vi "Phase 3 Sequence Struct.vi"() -> ()   [LabVIEW 2017]
uses:
  Classes/Sequence/SequenceSubvis/TestStepTypes.ctl
  Classes/Sequence/SequenceSubvis/PolarizationSelect.ctl
  Classes/Sequence/SequenceSubvis/RF Direction.ctl
  Classes/Sequence/SequenceSubvis/TestStep-StepType.ctl
panel:
  out "test sequence in the new struct":T3(array[cluster])=[{"StepType"=enum."Patch", "RF In/Out"=enum."Tx - RF In", "Module/Raster"=0, "Polarization"=enum."Vertical", "PhaseShift deg"=[], "Attenuation dB"=[], "Position"={"X mm"=204.374756, "Y mm"=144.119598, "Z mm"=0.0, "T deg"=1.0}, "Patch RF In/Out"=TRUE}, {"StepType"=enum."SweepTest", "RF In/Out"=enum."Tx - RF In", "Module/Raster"=0, "Polarization"=enum."Vertical", "PhaseShift deg"=[0.0, 5.625, 11.25, 16.875, 22.5, 28.125, 33.75, 39.375, 45.0], "Attenuation dB"=[5.5], "Position"={"X mm"=204.374756, "Y mm"=144.119598, "Z mm"=0.0, "T deg"=1.0}, "Patch RF In/Out"=FALSE}, {"StepType"=enum."Patch", "RF In/Out"=enum."Tx - RF In", "Module/Raster"=0, "Polarization"=enum."Horizontal", "PhaseShift deg"=[], "Attenuation dB"=[], "Position"={"X mm"=204.374756, "Y mm"=144.119598, "Z mm"=0.0, "T deg"=1.0}, "Patch RF In/Out"=FALSE}, {"StepType"=enum."SweepTest", "RF In/Out"=enum."Tx - RF In", "Module/Raster"=0, "Polarization"=enum."Horizontal", "PhaseShift deg"=[0.0, 5.625, 11.25, 16.875, 22.5, 28.125, 33.75, 39.375, 45.0], "Attenuation dB"=[5.5], "Position"={"X mm"=204.374756, "Y mm"=144.119598, "Z mm"=0.0, "T deg"=1.0}, "Patch RF In/Out"=FALSE}, {"StepType"=enum."Patch", "RF In/Out"=enum."Tx - RF In", "Module/Raster"=1, "Polarization"=enum."Vertical", "PhaseShift deg"=[], "Attenuation dB"=[], "Position"={"X mm"=232.088571, "Y mm"=144.281169, "Z mm"=0.0, "T deg"=1.0}, "Patch RF In/Out"=FALSE}, {"StepType"=enum."SweepTest", "RF In/Out"=enum."Tx - RF In", "Module/Raster"=1, "Polarization"=enum."Vertical", "PhaseShift deg"=[90.0, 95.625, 101.25, 106.875, 112.5], "Attenuation dB"=[0.0, 0.5, 1.0, 1.5, 2.0, 2.5, 3.0, 3.5, 4.0, 4.5, 5.0, 5.5, 6.0, 6.5, 7.0, 7.5, 8.0, 8.5], "Position"={"X mm"=232.088571, "Y mm"=144.281169, "Z mm"=0.0, "T deg"=1.0}, "Patch RF In/Out"=FALSE}, {"StepType"=enum."Patch", "RF In/Out"=enum."Tx - RF In", "Module/Raster"=2, "Polarization"=enum."Vertical", "PhaseShift deg"=[], "Attenuation dB"=[], "Position"={"X mm"=259.802385, "Y mm"=144.442739, "Z mm"=0.0, "T deg"=1.0}, "Patch RF In/Out"=FALSE}, {"StepType"=enum."SweepTest", "RF In/Out"=enum."Tx - RF In", "Module/Raster"=2, "Polarization"=enum."Vertical", "PhaseShift deg"=[11.25, 16.875, 22.5, 28.125, 33.75, 39.375, 45.0, 50.625, 56.25, 61.875, 67.5, 73.125, 78.75, 84.375, 90.0, 95.625, 101.25, 106.875, 112.5], "Attenuation dB"=[0.0, 5.5, 7.0, 8.0, 9.0, 9.5], "Position"={"X mm"=259.802385, "Y mm"=144.442739, "Z mm"=0.0, "T deg"=1.0}, "Patch RF In/Out"=FALSE}, {"StepType"=enum."Patch", "RF In/Out"=enum."Tx - RF In", "Module/Raster"=15, "Polarization"=enum."Vertical", "PhaseShift deg"=[], "Attenuation dB"=[], "Position"={"X mm"=398.209889, "Y mm"=172.964406, "Z mm"=0.0, "T deg"=1.0}, "Patch RF In/Out"=FALSE}, {"StepType"=enum."SweepTest", "RF In/Out"=enum."Tx - RF In", "Module/Raster"=15, "Polarization"=enum."Vertical", "PhaseShift deg"=[0.0, 5.625, 11.25, 16.875, 22.5], "Attenuation dB"=[0.0, 0.5, 1.0, 1.5, 2.0], "Position"={"X mm"=398.209889, "Y mm"=172.964406, "Z mm"=0.0, "T deg"=1.0}, "Patch RF In/Out"=FALSE}, {"StepType"=enum."Patch", "RF In/Out"=enum."Tx - RF In", "Module/Raster"=17, "Polarization"=enum."Vertical", "PhaseShift deg"=[], "Attenuation dB"=[], "Position"={"X mm"=231.76543, "Y mm"=199.708798, "Z mm"=0.0, "T deg"=1.0}, "Patch RF In/Out"=FALSE}, {"StepType"=enum."SweepTest", "RF In/Out"=enum."Tx - RF In", "Module/Raster"=17, "Polarization"=enum."Vertical", "PhaseShift deg"=[0.0, 5.625], "Attenuation dB"=[0.0, 0.5], "Position"={"X mm"=231.76543, "Y mm"=199.708798, "Z mm"=0.0, "T deg"=1.0}, "Patch RF In/Out"=FALSE}, {"StepType"=enum."Patch", "RF In/Out"=enum."Tx - RF In", "Module/Raster"=21, "Polarization"=enum."Vertical", "PhaseShift deg"=[], "Attenuation dB"=[], "Position"={"X mm"=342.620689, "Y mm"=200.35508, "Z mm"=0.0, "T deg"=1.0}, "Patch RF In/Out"=FALSE}, {"StepType"=enum."SweepTest", "RF In/Out"=enum."Tx - RF In", "Module/Raster"=21, "Polarization"=enum."Vertical", "PhaseShift deg"=[0.0], "Attenuation dB"=[0.0], "Position"={"X mm"=342.620689, "Y mm"=200.35508, "Z mm"=0.0, "T deg"=1.0}, "Patch RF In/Out"=FALSE}, {"StepType"=enum."Patch", "RF In/Out"=enum."Tx - RF In", "Module/Raster"=23, "Polarization"=enum."Vertical", "PhaseShift deg"=[], "Attenuation dB"=[], "Position"={"X mm"=398.048318, "Y mm"=200.678221, "Z mm"=0.0, "T deg"=1.0}, "Patch RF In/Out"=FALSE}, {"StepType"=enum."SweepTest", "RF In/Out"=enum."Tx - RF In", "Module/Raster"=23, "Polarization"=enum."Vertical", "PhaseShift deg"=[0.0], "Attenuation dB"=[0.0], "Position"={"X mm"=398.048318, "Y mm"=200.678221, "Z mm"=0.0, "T deg"=1.0}, "Patch RF In/Out"=FALSE}, {"StepType"=enum."Patch", "RF In/Out"=enum."Tx - RF In", "Module/Raster"=24, "Polarization"=enum."Vertical", "PhaseShift deg"=[], "Attenuation dB"=[], "Position"={"X mm"=203.890045, "Y mm"=227.261043, "Z mm"=0.0, "T deg"=1.0}, "Patch RF In/Out"=FALSE}, {"StepType"=enum."SweepTest", "RF In/Out"=enum."Tx - RF In", "Module/Raster"=24, "Polarization"=enum."Vertical", "PhaseShift deg"=[0.0, 5.625, 11.25], "Attenuation dB"=[0.0], "Position"={"X mm"=203.890045, "Y mm"=227.261043, "Z mm"=0.0, "T deg"=1.0}, "Patch RF In/Out"=FALSE}, {"StepType"=enum."Patch", "RF In/Out"=enum."Tx - RF In", "Module/Raster"=25, "Polarization"=enum."Vertical", "PhaseShift deg"=[], "Attenuation dB"=[], "Position"={"X mm"=231.603859, "Y mm"=227.422613, "Z mm"=0.0, "T deg"=1.0}, "Patch RF In/Out"=FALSE}, {"StepType"=enum."SweepTest", "RF In/Out"=enum."Tx - RF In", "Module/Raster"=25, "Polarization"=enum."Vertical", "PhaseShift deg"=[0.0], "Attenuation dB"=[0.0], "Position"={"X mm"=231.603859, "Y mm"=227.422613, "Z mm"=0.0, "T deg"=1.0}, "Patch RF In/Out"=FALSE}, {"StepType"=enum."Patch", "RF In/Out"=enum."Tx - RF In", "Module/Raster"=31, "Polarization"=enum."Vertical", "PhaseShift deg"=[], "Attenuation dB"=[], "Position"={"X mm"=397.886748, "Y mm"=228.392036, "Z mm"=0.0, "T deg"=1.0}, "Patch RF In/Out"=FALSE}, {"StepType"=enum."SweepTest", "RF In/Out"=enum."Tx - RF In", "Module/Raster"=31, "Polarization"=enum."Vertical", "PhaseShift deg"=[0.0, 5.625], "Attenuation dB"=[0.0], "Position"={"X mm"=397.886748, "Y mm"=228.392036, "Z mm"=0.0, "T deg"=1.0}, "Patch RF In/Out"=FALSE}, {"StepType"=enum."Patch", "RF In/Out"=enum."Tx - RF In", "Module/Raster"=31, "Polarization"=enum."Horizontal", "PhaseShift deg"=[], "Attenuation dB"=[], "Position"={"X mm"=397.886748, "Y mm"=228.392036, "Z mm"=0.0, "T deg"=1.0}, "Patch RF In/Out"=FALSE}, {"StepType"=enum."SweepTest", "RF In/Out"=enum."Tx - RF In", "Module/Raster"=31, "Polarization"=enum."Horizontal", "PhaseShift deg"=[0.0, 5.625], "Attenuation dB"=[0.0], "Position"={"X mm"=397.886748, "Y mm"=228.392036, "Z mm"=0.0, "T deg"=1.0}, "Patch RF In/Out"=FALSE}, {"StepType"=enum."Patch", "RF In/Out"=enum."Tx - RF In", "Module/Raster"=39, "Polarization"=enum."Vertical", "PhaseShift deg"=[], "Attenuation dB"=[], "Position"={"X mm"=397.725177, "Y mm"=256.10585, "Z mm"=0.0, "T deg"=1.0}, "Patch RF In/Out"=FALSE}, {"StepType"=enum."SweepTest", "RF In/Out"=enum."Tx - RF In", "Module/Raster"=39, "Polarization"=enum."Vertical", "PhaseShift deg"=[0.0], "Attenuation dB"=[0.0], "Position"={"X mm"=397.725177, "Y mm"=256.10585, "Z mm"=0.0, "T deg"=1.0}, "Patch RF In/Out"=FALSE}, {"StepType"=enum."Patch", "RF In/Out"=enum."Tx - RF In", "Module/Raster"=44, "Polarization"=enum."Vertical", "PhaseShift deg"=[], "Attenuation dB"=[], "Position"={"X mm"=314.422163, "Y mm"=283.334954, "Z mm"=0.0, "T deg"=1.0}, "Patch RF In/Out"=FALSE}, {"StepType"=enum."SweepTest", "RF In/Out"=enum."Tx - RF In", "Module/Raster"=44, "Polarization"=enum."Vertical", "PhaseShift deg"=[0.0, 5.625], "Attenuation dB"=[0.0, 0.5], "Position"={"X mm"=314.422163, "Y mm"=283.334954, "Z mm"=0.0, "T deg"=1.0}, "Patch RF In/Out"=FALSE}, {"StepType"=enum."Patch", "RF In/Out"=enum."Tx - RF In", "Module/Raster"=45, "Polarization"=enum."Vertical", "PhaseShift deg"=[], "Attenuation dB"=[], "Position"={"X mm"=342.135977, "Y mm"=283.496524, "Z mm"=0.0, "T deg"=1.0}, "Patch RF In/Out"=FALSE}, {"StepType"=enum."SweepTest", "RF In/Out"=enum."Tx - RF In", "Module/Raster"=45, "Polarization"=enum."Vertical", "PhaseShift deg"=[0.0], "Attenuation dB"=[0.0], "Position"={"X mm"=342.135977, "Y mm"=283.496524, "Z mm"=0.0, "T deg"=1.0}, "Patch RF In/Out"=FALSE}, {"StepType"=enum."Patch", "RF In/Out"=enum."Tx - RF In", "Module/Raster"=46, "Polarization"=enum."Vertical", "PhaseShift deg"=[], "Attenuation dB"=[], "Position"={"X mm"=369.849792, "Y mm"=283.658095, "Z mm"=0.0, "T deg"=1.0}, "Patch RF In/Out"=FALSE}, {"StepType"=enum."SweepTest", "RF In/Out"=enum."Tx - RF In", "Module/Raster"=46, "Polarization"=enum."Vertical", "PhaseShift deg"=[0.0, 5.625], "Attenuation dB"=[0.0, 0.5], "Position"={"X mm"=369.849792, "Y mm"=283.658095, "Z mm"=0.0, "T deg"=1.0}, "Patch RF In/Out"=FALSE}, {"StepType"=enum."Patch", "RF In/Out"=enum."Tx - RF In", "Module/Raster"=47, "Polarization"=enum."Vertical", "PhaseShift deg"=[], "Attenuation dB"=[], "Position"={"X mm"=397.563607, "Y mm"=283.819665, "Z mm"=0.0, "T deg"=1.0}, "Patch RF In/Out"=FALSE}, {"StepType"=enum."SweepTest", "RF In/Out"=enum."Tx - RF In", "Module/Raster"=47, "Polarization"=enum."Vertical", "PhaseShift deg"=[0.0], "Attenuation dB"=[0.0], "Position"={"X mm"=397.563607, "Y mm"=283.819665, "Z mm"=0.0, "T deg"=1.0}, "Patch RF In/Out"=FALSE}, {"StepType"=enum."Patch", "RF In/Out"=enum."Tx - RF In", "Module/Raster"=48, "Polarization"=enum."Vertical", "PhaseShift deg"=[], "Attenuation dB"=[], "Position"={"X mm"=203.405333, "Y mm"=310.402487, "Z mm"=0.0, "T deg"=1.0}, "Patch RF In/Out"=FALSE}, {"StepType"=enum."SweepTest", "RF In/Out"=enum."Tx - RF In", "Module/Raster"=48, "Polarization"=enum."Vertical", "PhaseShift deg"=[28.125], "Attenuation dB"=[2.5], "Position"={"X mm"=203.405333, "Y mm"=310.402487, "Z mm"=0.0, "T deg"=1.0}, "Patch RF In/Out"=FALSE}, {"StepType"=enum."Patch", "RF In/Out"=enum."Tx - RF In", "Module/Raster"=48, "Polarization"=enum."Horizontal", "PhaseShift deg"=[], "Attenuation dB"=[], "Position"={"X mm"=203.405333, "Y mm"=310.402487, "Z mm"=0.0, "T deg"=1.0}, "Patch RF In/Out"=FALSE}, {"StepType"=enum."SweepTest", "RF In/Out"=enum."Tx - RF In", "Module/Raster"=48, "Polarization"=enum."Horizontal", "PhaseShift deg"=[28.125], "Attenuation dB"=[2.5], "Position"={"X mm"=203.405333, "Y mm"=310.402487, "Z mm"=0.0, "T deg"=1.0}, "Patch RF In/Out"=FALSE}, {"StepType"=enum."Patch", "RF In/Out"=enum."Tx - RF In", "Module/Raster"=55, "Polarization"=enum."Vertical", "PhaseShift deg"=[], "Attenuation dB"=[], "Position"={"X mm"=397.402037, "Y mm"=311.53348, "Z mm"=0.0, "T deg"=1.0}, "Patch RF In/Out"=FALSE}, {"StepType"=enum."SweepTest", "RF In/Out"=enum."Tx - RF In", "Module/Raster"=55, "Polarization"=enum."Vertical", "PhaseShift deg"=[0.0, 5.625, 11.25, 16.875, 22.5], "Attenuation dB"=[0.0, 0.5, 1.0], "Position"={"X mm"=397.402037, "Y mm"=311.53348, "Z mm"=0.0, "T deg"=1.0}, "Patch RF In/Out"=FALSE}, {"StepType"=enum."Patch", "RF In/Out"=enum."Tx - RF In", "Module/Raster"=59, "Polarization"=enum."Vertical", "PhaseShift deg"=[], "Attenuation dB"=[], "Position"={"X mm"=286.385207, "Y mm"=338.601013, "Z mm"=0.0, "T deg"=1.0}, "Patch RF In/Out"=FALSE}, {"StepType"=enum."SweepTest", "RF In/Out"=enum."Tx - RF In", "Module/Raster"=59, "Polarization"=enum."Vertical", "PhaseShift deg"=[0.0], "Attenuation dB"=[0.0], "Position"={"X mm"=286.385207, "Y mm"=338.601013, "Z mm"=0.0, "T deg"=1.0}, "Patch RF In/Out"=FALSE}, {"StepType"=enum."Patch", "RF In/Out"=enum."Tx - RF In", "Module/Raster"=59, "Polarization"=enum."Horizontal", "PhaseShift deg"=[], "Attenuation dB"=[], "Position"={"X mm"=286.385207, "Y mm"=338.601013, "Z mm"=0.0, "T deg"=1.0}, "Patch RF In/Out"=FALSE}, {"StepType"=enum."SweepTest", "RF In/Out"=enum."Tx - RF In", "Module/Raster"=59, "Polarization"=enum."Horizontal", "PhaseShift deg"=[0.0], "Attenuation dB"=[0.0], "Position"={"X mm"=286.385207, "Y mm"=338.601013, "Z mm"=0.0, "T deg"=1.0}, "Patch RF In/Out"=FALSE}, {"StepType"=enum."Patch", "RF In/Out"=enum."Tx - RF In", "Module/Raster"=62, "Polarization"=enum."Vertical", "PhaseShift deg"=[], "Attenuation dB"=[], "Position"={"X mm"=369.526651, "Y mm"=339.085724, "Z mm"=0.0, "T deg"=1.0}, "Patch RF In/Out"=FALSE}, {"StepType"=enum."SweepTest", "RF In/Out"=enum."Tx - RF In", "Module/Raster"=62, "Polarization"=enum."Vertical", "PhaseShift deg"=[0.0, 5.625, 11.25, 16.875, 22.5, 28.125], "Attenuation dB"=[0.0, 0.5, 1.0, 1.5, 2.0, 2.5], "Position"={"X mm"=369.526651, "Y mm"=339.085724, "Z mm"=0.0, "T deg"=1.0}, "Patch RF In/Out"=FALSE}, {"StepType"=enum."Patch", "RF In/Out"=enum."Tx - RF In", "Module/Raster"=63, "Polarization"=enum."Vertical", "PhaseShift deg"=[], "Attenuation dB"=[], "Position"={"X mm"=397.240466, "Y mm"=339.247295, "Z mm"=0.0, "T deg"=1.0}, "Patch RF In/Out"=FALSE}, {"StepType"=enum."SweepTest", "RF In/Out"=enum."Tx - RF In", "Module/Raster"=63, "Polarization"=enum."Vertical", "PhaseShift deg"=[0.0, 5.625, 11.25, 16.875, 22.5, 28.125], "Attenuation dB"=[0.0, 0.5, 1.0, 1.5, 2.0, 2.5], "Position"={"X mm"=397.240466, "Y mm"=339.247295, "Z mm"=0.0, "T deg"=1.0}, "Patch RF In/Out"=FALSE}, {"StepType"=enum."Patch", "RF In/Out"=enum."Rx - RF Out", "Module/Raster"=0, "Polarization"=enum."Vertical", "PhaseShift deg"=[], "Attenuation dB"=[], "Position"={"X mm"=204.374756, "Y mm"=144.119598, "Z mm"=0.0, "T deg"=1.0}, "Patch RF In/Out"=TRUE}, {"StepType"=enum."SweepTest", "RF In/Out"=enum."Rx - RF Out", "Module/Raster"=0, "Polarization"=enum."Vertical", "PhaseShift deg"=[0.0, 5.625, 11.25, 16.875, 22.5, 28.125, 33.75, 39.375, 45.0], "Attenuation dB"=[5.5], "Position"={"X mm"=204.374756, "Y mm"=144.119598, "Z mm"=0.0, "T deg"=1.0}, "Patch RF In/Out"=FALSE}, {"StepType"=enum."Patch", "RF In/Out"=enum."Rx - RF Out", "Module/Raster"=0, "Polarization"=enum."Horizontal", "PhaseShift deg"=[], "Attenuation dB"=[], "Position"={"X mm"=204.374756, "Y mm"=144.119598, "Z mm"=0.0, "T deg"=1.0}, "Patch RF In/Out"=FALSE}, {"StepType"=enum."SweepTest", "RF In/Out"=enum."Rx - RF Out", "Module/Raster"=0, "Polarization"=enum."Horizontal", "PhaseShift deg"=[0.0, 5.625, 11.25, 16.875, 22.5, 28.125, 33.75, 39.375, 45.0], "Attenuation dB"=[5.5], "Position"={"X mm"=204.374756, "Y mm"=144.119598, "Z mm"=0.0, "T deg"=1.0}, "Patch RF In/Out"=FALSE}, {"StepType"=enum."Patch", "RF In/Out"=enum."Rx - RF Out", "Module/Raster"=17, "Polarization"=enum."Horizontal", "PhaseShift deg"=[], "Attenuation dB"=[], "Position"={"X mm"=231.76543, "Y mm"=199.708798, "Z mm"=0.0, "T deg"=1.0}, "Patch RF In/Out"=FALSE}, {"StepType"=enum."SweepTest", "RF In/Out"=enum."Rx - RF Out", "Module/Raster"=17, "Polarization"=enum."Horizontal", "PhaseShift deg"=[0.0, 5.625], "Attenuation dB"=[0.0, 0.5], "Position"={"X mm"=231.76543, "Y mm"=199.708798, "Z mm"=0.0, "T deg"=1.0}, "Patch RF In/Out"=FALSE}, {"StepType"=enum."Patch", "RF In/Out"=enum."Rx - RF Out", "Module/Raster"=28, "Polarization"=enum."Vertical", "PhaseShift deg"=[], "Attenuation dB"=[], "Position"={"X mm"=314.745304, "Y mm"=227.907324, "Z mm"=0.0, "T deg"=1.0}, "Patch RF In/Out"=FALSE}, {"StepType"=enum."SweepTest", "RF In/Out"=enum."Rx - RF Out", "Module/Raster"=28, "Polarization"=enum."Vertical", "PhaseShift deg"=[0.0], "Attenuation dB"=[0.0], "Position"={"X mm"=314.745304, "Y mm"=227.907324, "Z mm"=0.0, "T deg"=1.0}, "Patch RF In/Out"=FALSE}, {"StepType"=enum."Patch", "RF In/Out"=enum."Rx - RF Out", "Module/Raster"=28, "Polarization"=enum."Horizontal", "PhaseShift deg"=[], "Attenuation dB"=[], "Position"={"X mm"=314.745304, "Y mm"=227.907324, "Z mm"=0.0, "T deg"=1.0}, "Patch RF In/Out"=FALSE}, {"StepType"=enum."SweepTest", "RF In/Out"=enum."Rx - RF Out", "Module/Raster"=28, "Polarization"=enum."Horizontal", "PhaseShift deg"=[0.0], "Attenuation dB"=[0.0], "Position"={"X mm"=314.745304, "Y mm"=227.907324, "Z mm"=0.0, "T deg"=1.0}, "Patch RF In/Out"=FALSE}, {"StepType"=enum."Patch", "RF In/Out"=enum."Rx - RF Out", "Module/Raster"=31, "Polarization"=enum."Vertical", "PhaseShift deg"=[], "Attenuation dB"=[], "Position"={"X mm"=397.886748, "Y mm"=228.392036, "Z mm"=0.0, "T deg"=1.0}, "Patch RF In/Out"=FALSE}, {"StepType"=enum."SweepTest", "RF In/Out"=enum."Rx - RF Out", "Module/Raster"=31, "Polarization"=enum."Vertical", "PhaseShift deg"=[0.0, 5.625], "Attenuation dB"=[0.0], "Position"={"X mm"=397.886748, "Y mm"=228.392036, "Z mm"=0.0, "T deg"=1.0}, "Patch RF In/Out"=FALSE}, {"StepType"=enum."Patch", "RF In/Out"=enum."Rx - RF Out", "Module/Raster"=31, "Polarization"=enum."Horizontal", "PhaseShift deg"=[], "Attenuation dB"=[], "Position"={"X mm"=397.886748, "Y mm"=228.392036, "Z mm"=0.0, "T deg"=1.0}, "Patch RF In/Out"=FALSE}, {"StepType"=enum."SweepTest", "RF In/Out"=enum."Rx - RF Out", "Module/Raster"=31, "Polarization"=enum."Horizontal", "PhaseShift deg"=[0.0, 5.625], "Attenuation dB"=[0.0], "Position"={"X mm"=397.886748, "Y mm"=228.392036, "Z mm"=0.0, "T deg"=1.0}, "Patch RF In/Out"=FALSE}, {"StepType"=enum."Patch", "RF In/Out"=enum."Rx - RF Out", "Module/Raster"=36, "Polarization"=enum."Vertical", "PhaseShift deg"=[], "Attenuation dB"=[], "Position"={"X mm"=314.583733, "Y mm"=255.621139, "Z mm"=0.0, "T deg"=1.0}, "Patch RF In/Out"=FALSE}, {"StepType"=enum."SweepTest", "RF In/Out"=enum."Rx - RF Out", "Module/Raster"=36, "Polarization"=enum."Vertical", "PhaseShift deg"=[28.125, 33.75, 39.375, 45.0, 50.625], "Attenuation dB"=[5.0, 5.5, 6.0, 6.5, 7.0], "Position"={"X mm"=314.583733, "Y mm"=255.621139, "Z mm"=0.0, "T deg"=1.0}, "Patch RF In/Out"=FALSE}, {"StepType"=enum."Patch", "RF In/Out"=enum."Rx - RF Out", "Module/Raster"=36, "Polarization"=enum."Horizontal", "PhaseShift deg"=[], "Attenuation dB"=[], "Position"={"X mm"=314.583733, "Y mm"=255.621139, "Z mm"=0.0, "T deg"=1.0}, "Patch RF In/Out"=FALSE}, {"StepType"=enum."SweepTest", "RF In/Out"=enum."Rx - RF Out", "Module/Raster"=36, "Polarization"=enum."Horizontal", "PhaseShift deg"=[28.125, 33.75, 39.375, 45.0, 50.625], "Attenuation dB"=[5.0, 5.5, 6.0, 6.5, 7.0], "Position"={"X mm"=314.583733, "Y mm"=255.621139, "Z mm"=0.0, "T deg"=1.0}, "Patch RF In/Out"=FALSE}, {"StepType"=enum."Patch", "RF In/Out"=enum."Rx - RF Out", "Module/Raster"=48, "Polarization"=enum."Vertical", "PhaseShift deg"=[], "Attenuation dB"=[], "Position"={"X mm"=203.405333, "Y mm"=310.402487, "Z mm"=0.0, "T deg"=1.0}, "Patch RF In/Out"=FALSE}, {"StepType"=enum."SweepTest", "RF In/Out"=enum."Rx - RF Out", "Module/Raster"=48, "Polarization"=enum."Vertical", "PhaseShift deg"=[28.125], "Attenuation dB"=[2.5], "Position"={"X mm"=203.405333, "Y mm"=310.402487, "Z mm"=0.0, "T deg"=1.0}, "Patch RF In/Out"=FALSE}, {"StepType"=enum."Patch", "RF In/Out"=enum."Rx - RF Out", "Module/Raster"=48, "Polarization"=enum."Horizontal", "PhaseShift deg"=[], "Attenuation dB"=[], "Position"={"X mm"=203.405333, "Y mm"=310.402487, "Z mm"=0.0, "T deg"=1.0}, "Patch RF In/Out"=FALSE}, {"StepType"=enum."SweepTest", "RF In/Out"=enum."Rx - RF Out", "Module/Raster"=48, "Polarization"=enum."Horizontal", "PhaseShift deg"=[28.125], "Attenuation dB"=[2.5], "Position"={"X mm"=203.405333, "Y mm"=310.402487, "Z mm"=0.0, "T deg"=1.0}, "Patch RF In/Out"=FALSE}, {"StepType"=enum."Patch", "RF In/Out"=enum."Rx - RF Out", "Module/Raster"=59, "Polarization"=enum."Vertical", "PhaseShift deg"=[], "Attenuation dB"=[], "Position"={"X mm"=286.385207, "Y mm"=338.601013, "Z mm"=0.0, "T deg"=1.0}, "Patch RF In/Out"=FALSE}, {"StepType"=enum."SweepTest", "RF In/Out"=enum."Rx - RF Out", "Module/Raster"=59, "Polarization"=enum."Vertical", "PhaseShift deg"=[0.0], "Attenuation dB"=[0.0], "Position"={"X mm"=286.385207, "Y mm"=338.601013, "Z mm"=0.0, "T deg"=1.0}, "Patch RF In/Out"=FALSE}, {"StepType"=enum."Patch", "RF In/Out"=enum."Rx - RF Out", "Module/Raster"=59, "Polarization"=enum."Horizontal", "PhaseShift deg"=[], "Attenuation dB"=[], "Position"={"X mm"=286.385207, "Y mm"=338.601013, "Z mm"=0.0, "T deg"=1.0}, "Patch RF In/Out"=FALSE}, {"StepType"=enum."SweepTest", "RF In/Out"=enum."Rx - RF Out", "Module/Raster"=59, "Polarization"=enum."Horizontal", "PhaseShift deg"=[0.0], "Attenuation dB"=[0.0], "Position"={"X mm"=286.385207, "Y mm"=338.601013, "Z mm"=0.0, "T deg"=1.0}, "Patch RF In/Out"=FALSE}, {"StepType"=enum."Patch", "RF In/Out"=enum."Rx - RF Out", "Module/Raster"=62, "Polarization"=enum."Vertical", "PhaseShift deg"=[], "Attenuation dB"=[], "Position"={"X mm"=369.526651, "Y mm"=339.085724, "Z mm"=0.0, "T deg"=1.0}, "Patch RF In/Out"=FALSE}, {"StepType"=enum."SweepTest", "RF In/Out"=enum."Rx - RF Out", "Module/Raster"=62, "Polarization"=enum."Vertical", "PhaseShift deg"=[0.0, 5.625, 11.25, 16.875, 22.5, 28.125], "Attenuation dB"=[0.0, 0.5, 1.0, 1.5, 2.0, 2.5], "Position"={"X mm"=369.526651, "Y mm"=339.085724, "Z mm"=0.0, "T deg"=1.0}, "Patch RF In/Out"=FALSE}, {"StepType"=enum."Patch", "RF In/Out"=enum."Rx - RF Out", "Module/Raster"=63, "Polarization"=enum."Vertical", "PhaseShift deg"=[], "Attenuation dB"=[], "Position"={"X mm"=397.240466, "Y mm"=339.247295, "Z mm"=0.0, "T deg"=1.0}, "Patch RF In/Out"=FALSE}, {"StepType"=enum."SweepTest", "RF In/Out"=enum."Rx - RF Out", "Module/Raster"=63, "Polarization"=enum."Vertical", "PhaseShift deg"=[0.0, 5.625, 11.25, 16.875, 22.5, 28.125], "Attenuation dB"=[0.0, 0.5, 1.0, 1.5, 2.0, 2.5], "Position"={"X mm"=397.240466, "Y mm"=339.247295, "Z mm"=0.0, "T deg"=1.0}, "Patch RF In/Out"=FALSE}, {"StepType"=enum."Finish", "RF In/Out"=enum."Tx - RF In", "Module/Raster"=0, "Polarization"=enum."Vertical", "PhaseShift deg"=[], "Attenuation dB"=[], "Position"={"X mm"=204.374756, "Y mm"=144.119598, "Z mm"=0.0, "T deg"=1.0}, "Patch RF In/Out"=FALSE}]
  out "TestSequence New":T3(array[cluster])
  in  "Motion":bool
  in  "from Raster Test File":T4
  in  "Raster":bool
  in  "TestSequence":T5[](array[typedef])=[{"RF In/Out"=enum."Tx - RF In", "TR Module 0-7"=0, "Polarization"=enum."Vertical", "PhaseShift deg"=[], "Attenuation dB"=[], "StepType"=enum."NewConnection"}, {"RF In/Out"=enum."Tx - RF In", "TR Module 0-7"=0, "Polarization"=enum."Vertical", "PhaseShift deg"=[0.0, 5.625, 11.25, 16.875, 22.5, 28.125, 33.75, 39.375, 45.0], "Attenuation dB"=[5.5], "StepType"=enum."SweepTest"}, {"RF In/Out"=enum."Tx - RF In", "TR Module 0-7"=0, "Polarization"=enum."Horizontal", "PhaseShift deg"=[], "Attenuation dB"=[], "StepType"=enum."NewConnection"}, {"RF In/Out"=enum."Tx - RF In", "TR Module 0-7"=0, "Polarization"=enum."Horizontal", "PhaseShift deg"=[0.0, 5.625, 11.25, 16.875, 22.5, 28.125, 33.75, 39.375, 45.0], "Attenuation dB"=[5.5], "StepType"=enum."SweepTest"}, {"RF In/Out"=enum."Tx - RF In", "TR Module 0-7"=1, "Polarization"=enum."Vertical", "PhaseShift deg"=[], "Attenuation dB"=[], "StepType"=enum."NewConnection"}, {"RF In/Out"=enum."Tx - RF In", "TR Module 0-7"=1, "Polarization"=enum."Vertical", "PhaseShift deg"=[90.0, 95.625, 101.25, 106.875, 112.5], "Attenuation dB"=[0.0, 0.5, 1.0, 1.5, 2.0, 2.5, 3.0, 3.5, 4.0, 4.5, 5.0, 5.5, 6.0, 6.5, 7.0, 7.5, 8.0, 8.5], "StepType"=enum."SweepTest"}, {"RF In/Out"=enum."Tx - RF In", "TR Module 0-7"=2, "Polarization"=enum."Vertical", "PhaseShift deg"=[], "Attenuation dB"=[], "StepType"=enum."NewConnection"}, {"RF In/Out"=enum."Tx - RF In", "TR Module 0-7"=2, "Polarization"=enum."Vertical", "PhaseShift deg"=[11.25, 16.875, 22.5, 28.125, 33.75, 39.375, 45.0, 50.625, 56.25, 61.875, 67.5, 73.125, 78.75, 84.375, 90.0, 95.625, 101.25, 106.875, 112.5], "Attenuation dB"=[0.0, 5.5, 7.0, 8.0, 9.0, 9.5], "StepType"=enum."SweepTest"}, {"RF In/Out"=enum."Tx - RF In", "TR Module 0-7"=15, "Polarization"=enum."Vertical", "PhaseShift deg"=[], "Attenuation dB"=[], "StepType"=enum."NewConnection"}, {"RF In/Out"=enum."Tx - RF In", "TR Module 0-7"=15, "Polarization"=enum."Vertical", "PhaseShift deg"=[0.0, 5.625, 11.25, 16.875, 22.5], "Attenuation dB"=[0.0, 0.5, 1.0, 1.5, 2.0], "StepType"=enum."SweepTest"}, {"RF In/Out"=enum."Tx - RF In", "TR Module 0-7"=17, "Polarization"=enum."Vertical", "PhaseShift deg"=[], "Attenuation dB"=[], "StepType"=enum."NewConnection"}, {"RF In/Out"=enum."Tx - RF In", "TR Module 0-7"=17, "Polarization"=enum."Vertical", "PhaseShift deg"=[0.0, 5.625], "Attenuation dB"=[0.0, 0.5], "StepType"=enum."SweepTest"}, {"RF In/Out"=enum."Tx - RF In", "TR Module 0-7"=21, "Polarization"=enum."Vertical", "PhaseShift deg"=[], "Attenuation dB"=[], "StepType"=enum."NewConnection"}, {"RF In/Out"=enum."Tx - RF In", "TR Module 0-7"=21, "Polarization"=enum."Vertical", "PhaseShift deg"=[0.0], "Attenuation dB"=[0.0], "StepType"=enum."SweepTest"}, {"RF In/Out"=enum."Tx - RF In", "TR Module 0-7"=23, "Polarization"=enum."Vertical", "PhaseShift deg"=[], "Attenuation dB"=[], "StepType"=enum."NewConnection"}, {"RF In/Out"=enum."Tx - RF In", "TR Module 0-7"=23, "Polarization"=enum."Vertical", "PhaseShift deg"=[0.0], "Attenuation dB"=[0.0], "StepType"=enum."SweepTest"}, {"RF In/Out"=enum."Tx - RF In", "TR Module 0-7"=24, "Polarization"=enum."Vertical", "PhaseShift deg"=[], "Attenuation dB"=[], "StepType"=enum."NewConnection"}, {"RF In/Out"=enum."Tx - RF In", "TR Module 0-7"=24, "Polarization"=enum."Vertical", "PhaseShift deg"=[0.0, 5.625, 11.25], "Attenuation dB"=[0.0], "StepType"=enum."SweepTest"}, {"RF In/Out"=enum."Tx - RF In", "TR Module 0-7"=25, "Polarization"=enum."Vertical", "PhaseShift deg"=[], "Attenuation dB"=[], "StepType"=enum."NewConnection"}, {"RF In/Out"=enum."Tx - RF In", "TR Module 0-7"=25, "Polarization"=enum."Vertical", "PhaseShift deg"=[0.0], "Attenuation dB"=[0.0], "StepType"=enum."SweepTest"}, {"RF In/Out"=enum."Tx - RF In", "TR Module 0-7"=31, "Polarization"=enum."Vertical", "PhaseShift deg"=[], "Attenuation dB"=[], "StepType"=enum."NewConnection"}, {"RF In/Out"=enum."Tx - RF In", "TR Module 0-7"=31, "Polarization"=enum."Vertical", "PhaseShift deg"=[0.0, 5.625], "Attenuation dB"=[0.0], "StepType"=enum."SweepTest"}, {"RF In/Out"=enum."Tx - RF In", "TR Module 0-7"=31, "Polarization"=enum."Horizontal", "PhaseShift deg"=[], "Attenuation dB"=[], "StepType"=enum."NewConnection"}, {"RF In/Out"=enum."Tx - RF In", "TR Module 0-7"=31, "Polarization"=enum."Horizontal", "PhaseShift deg"=[0.0, 5.625], "Attenuation dB"=[0.0], "StepType"=enum."SweepTest"}, {"RF In/Out"=enum."Tx - RF In", "TR Module 0-7"=39, "Polarization"=enum."Vertical", "PhaseShift deg"=[], "Attenuation dB"=[], "StepType"=enum."NewConnection"}, {"RF In/Out"=enum."Tx - RF In", "TR Module 0-7"=39, "Polarization"=enum."Vertical", "PhaseShift deg"=[0.0], "Attenuation dB"=[0.0], "StepType"=enum."SweepTest"}, {"RF In/Out"=enum."Tx - RF In", "TR Module 0-7"=44, "Polarization"=enum."Vertical", "PhaseShift deg"=[], "Attenuation dB"=[], "StepType"=enum."NewConnection"}, {"RF In/Out"=enum."Tx - RF In", "TR Module 0-7"=44, "Polarization"=enum."Vertical", "PhaseShift deg"=[0.0, 5.625], "Attenuation dB"=[0.0, 0.5], "StepType"=enum."SweepTest"}, {"RF In/Out"=enum."Tx - RF In", "TR Module 0-7"=45, "Polarization"=enum."Vertical", "PhaseShift deg"=[], "Attenuation dB"=[], "StepType"=enum."NewConnection"}, {"RF In/Out"=enum."Tx - RF In", "TR Module 0-7"=45, "Polarization"=enum."Vertical", "PhaseShift deg"=[0.0], "Attenuation dB"=[0.0], "StepType"=enum."SweepTest"}, {"RF In/Out"=enum."Tx - RF In", "TR Module 0-7"=46, "Polarization"=enum."Vertical", "PhaseShift deg"=[], "Attenuation dB"=[], "StepType"=enum."NewConnection"}, {"RF In/Out"=enum."Tx - RF In", "TR Module 0-7"=46, "Polarization"=enum."Vertical", "PhaseShift deg"=[0.0, 5.625], "Attenuation dB"=[0.0, 0.5], "StepType"=enum."SweepTest"}, {"RF In/Out"=enum."Tx - RF In", "TR Module 0-7"=47, "Polarization"=enum."Vertical", "PhaseShift deg"=[], "Attenuation dB"=[], "StepType"=enum."NewConnection"}, {"RF In/Out"=enum."Tx - RF In", "TR Module 0-7"=47, "Polarization"=enum."Vertical", "PhaseShift deg"=[0.0], "Attenuation dB"=[0.0], "StepType"=enum."SweepTest"}, {"RF In/Out"=enum."Tx - RF In", "TR Module 0-7"=48, "Polarization"=enum."Vertical", "PhaseShift deg"=[], "Attenuation dB"=[], "StepType"=enum."NewConnection"}, {"RF In/Out"=enum."Tx - RF In", "TR Module 0-7"=48, "Polarization"=enum."Vertical", "PhaseShift deg"=[28.125], "Attenuation dB"=[2.5], "StepType"=enum."SweepTest"}, {"RF In/Out"=enum."Tx - RF In", "TR Module 0-7"=48, "Polarization"=enum."Horizontal", "PhaseShift deg"=[], "Attenuation dB"=[], "StepType"=enum."NewConnection"}, {"RF In/Out"=enum."Tx - RF In", "TR Module 0-7"=48, "Polarization"=enum."Horizontal", "PhaseShift deg"=[28.125], "Attenuation dB"=[2.5], "StepType"=enum."SweepTest"}, {"RF In/Out"=enum."Tx - RF In", "TR Module 0-7"=55, "Polarization"=enum."Vertical", "PhaseShift deg"=[], "Attenuation dB"=[], "StepType"=enum."NewConnection"}, {"RF In/Out"=enum."Tx - RF In", "TR Module 0-7"=55, "Polarization"=enum."Vertical", "PhaseShift deg"=[0.0, 5.625, 11.25, 16.875, 22.5], "Attenuation dB"=[0.0, 0.5, 1.0], "StepType"=enum."SweepTest"}, {"RF In/Out"=enum."Tx - RF In", "TR Module 0-7"=59, "Polarization"=enum."Vertical", "PhaseShift deg"=[], "Attenuation dB"=[], "StepType"=enum."NewConnection"}, {"RF In/Out"=enum."Tx - RF In", "TR Module 0-7"=59, "Polarization"=enum."Vertical", "PhaseShift deg"=[0.0], "Attenuation dB"=[0.0], "StepType"=enum."SweepTest"}, {"RF In/Out"=enum."Tx - RF In", "TR Module 0-7"=59, "Polarization"=enum."Horizontal", "PhaseShift deg"=[], "Attenuation dB"=[], "StepType"=enum."NewConnection"}, {"RF In/Out"=enum."Tx - RF In", "TR Module 0-7"=59, "Polarization"=enum."Horizontal", "PhaseShift deg"=[0.0], "Attenuation dB"=[0.0], "StepType"=enum."SweepTest"}, {"RF In/Out"=enum."Tx - RF In", "TR Module 0-7"=62, "Polarization"=enum."Vertical", "PhaseShift deg"=[], "Attenuation dB"=[], "StepType"=enum."NewConnection"}, {"RF In/Out"=enum."Tx - RF In", "TR Module 0-7"=62, "Polarization"=enum."Vertical", "PhaseShift deg"=[0.0, 5.625, 11.25, 16.875, 22.5, 28.125], "Attenuation dB"=[0.0, 0.5, 1.0, 1.5, 2.0, 2.5], "StepType"=enum."SweepTest"}, {"RF In/Out"=enum."Tx - RF In", "TR Module 0-7"=63, "Polarization"=enum."Vertical", "PhaseShift deg"=[], "Attenuation dB"=[], "StepType"=enum."NewConnection"}, {"RF In/Out"=enum."Tx - RF In", "TR Module 0-7"=63, "Polarization"=enum."Vertical", "PhaseShift deg"=[0.0, 5.625, 11.25, 16.875, 22.5, 28.125], "Attenuation dB"=[0.0, 0.5, 1.0, 1.5, 2.0, 2.5], "StepType"=enum."SweepTest"}, {"RF In/Out"=enum."Rx - RF Out", "TR Module 0-7"=0, "Polarization"=enum."Vertical", "PhaseShift deg"=[], "Attenuation dB"=[], "StepType"=enum."NewConnection"}, {"RF In/Out"=enum."Rx - RF Out", "TR Module 0-7"=0, "Polarization"=enum."Vertical", "PhaseShift deg"=[0.0, 5.625, 11.25, 16.875, 22.5, 28.125, 33.75, 39.375, 45.0], "Attenuation dB"=[5.5], "StepType"=enum."SweepTest"}, {"RF In/Out"=enum."Rx - RF Out", "TR Module 0-7"=0, "Polarization"=enum."Horizontal", "PhaseShift deg"=[], "Attenuation dB"=[], "StepType"=enum."NewConnection"}, {"RF In/Out"=enum."Rx - RF Out", "TR Module 0-7"=0, "Polarization"=enum."Horizontal", "PhaseShift deg"=[0.0, 5.625, 11.25, 16.875, 22.5, 28.125, 33.75, 39.375, 45.0], "Attenuation dB"=[5.5], "StepType"=enum."SweepTest"}, {"RF In/Out"=enum."Rx - RF Out", "TR Module 0-7"=17, "Polarization"=enum."Horizontal", "PhaseShift deg"=[], "Attenuation dB"=[], "StepType"=enum."NewConnection"}, {"RF In/Out"=enum."Rx - RF Out", "TR Module 0-7"=17, "Polarization"=enum."Horizontal", "PhaseShift deg"=[0.0, 5.625], "Attenuation dB"=[0.0, 0.5], "StepType"=enum."SweepTest"}, {"RF In/Out"=enum."Rx - RF Out", "TR Module 0-7"=28, "Polarization"=enum."Vertical", "PhaseShift deg"=[], "Attenuation dB"=[], "StepType"=enum."NewConnection"}, {"RF In/Out"=enum."Rx - RF Out", "TR Module 0-7"=28, "Polarization"=enum."Vertical", "PhaseShift deg"=[0.0], "Attenuation dB"=[0.0], "StepType"=enum."SweepTest"}, {"RF In/Out"=enum."Rx - RF Out", "TR Module 0-7"=28, "Polarization"=enum."Horizontal", "PhaseShift deg"=[], "Attenuation dB"=[], "StepType"=enum."NewConnection"}, {"RF In/Out"=enum."Rx - RF Out", "TR Module 0-7"=28, "Polarization"=enum."Horizontal", "PhaseShift deg"=[0.0], "Attenuation dB"=[0.0], "StepType"=enum."SweepTest"}, {"RF In/Out"=enum."Rx - RF Out", "TR Module 0-7"=31, "Polarization"=enum."Vertical", "PhaseShift deg"=[], "Attenuation dB"=[], "StepType"=enum."NewConnection"}, {"RF In/Out"=enum."Rx - RF Out", "TR Module 0-7"=31, "Polarization"=enum."Vertical", "PhaseShift deg"=[0.0, 5.625], "Attenuation dB"=[0.0], "StepType"=enum."SweepTest"}, {"RF In/Out"=enum."Rx - RF Out", "TR Module 0-7"=31, "Polarization"=enum."Horizontal", "PhaseShift deg"=[], "Attenuation dB"=[], "StepType"=enum."NewConnection"}, {"RF In/Out"=enum."Rx - RF Out", "TR Module 0-7"=31, "Polarization"=enum."Horizontal", "PhaseShift deg"=[0.0, 5.625], "Attenuation dB"=[0.0], "StepType"=enum."SweepTest"}, {"RF In/Out"=enum."Rx - RF Out", "TR Module 0-7"=36, "Polarization"=enum."Vertical", "PhaseShift deg"=[], "Attenuation dB"=[], "StepType"=enum."NewConnection"}, {"RF In/Out"=enum."Rx - RF Out", "TR Module 0-7"=36, "Polarization"=enum."Vertical", "PhaseShift deg"=[28.125, 33.75, 39.375, 45.0, 50.625], "Attenuation dB"=[5.0, 5.5, 6.0, 6.5, 7.0], "StepType"=enum."SweepTest"}, {"RF In/Out"=enum."Rx - RF Out", "TR Module 0-7"=36, "Polarization"=enum."Horizontal", "PhaseShift deg"=[], "Attenuation dB"=[], "StepType"=enum."NewConnection"}, {"RF In/Out"=enum."Rx - RF Out", "TR Module 0-7"=36, "Polarization"=enum."Horizontal", "PhaseShift deg"=[28.125, 33.75, 39.375, 45.0, 50.625], "Attenuation dB"=[5.0, 5.5, 6.0, 6.5, 7.0], "StepType"=enum."SweepTest"}, {"RF In/Out"=enum."Rx - RF Out", "TR Module 0-7"=48, "Polarization"=enum."Vertical", "PhaseShift deg"=[], "Attenuation dB"=[], "StepType"=enum."NewConnection"}, {"RF In/Out"=enum."Rx - RF Out", "TR Module 0-7"=48, "Polarization"=enum."Vertical", "PhaseShift deg"=[28.125], "Attenuation dB"=[2.5], "StepType"=enum."SweepTest"}, {"RF In/Out"=enum."Rx - RF Out", "TR Module 0-7"=48, "Polarization"=enum."Horizontal", "PhaseShift deg"=[], "Attenuation dB"=[], "StepType"=enum."NewConnection"}, {"RF In/Out"=enum."Rx - RF Out", "TR Module 0-7"=48, "Polarization"=enum."Horizontal", "PhaseShift deg"=[28.125], "Attenuation dB"=[2.5], "StepType"=enum."SweepTest"}, {"RF In/Out"=enum."Rx - RF Out", "TR Module 0-7"=59, "Polarization"=enum."Vertical", "PhaseShift deg"=[], "Attenuation dB"=[], "StepType"=enum."NewConnection"}, {"RF In/Out"=enum."Rx - RF Out", "TR Module 0-7"=59, "Polarization"=enum."Vertical", "PhaseShift deg"=[0.0], "Attenuation dB"=[0.0], "StepType"=enum."SweepTest"}, {"RF In/Out"=enum."Rx - RF Out", "TR Module 0-7"=59, "Polarization"=enum."Horizontal", "PhaseShift deg"=[], "Attenuation dB"=[], "StepType"=enum."NewConnection"}, {"RF In/Out"=enum."Rx - RF Out", "TR Module 0-7"=59, "Polarization"=enum."Horizontal", "PhaseShift deg"=[0.0], "Attenuation dB"=[0.0], "StepType"=enum."SweepTest"}, {"RF In/Out"=enum."Rx - RF Out", "TR Module 0-7"=62, "Polarization"=enum."Vertical", "PhaseShift deg"=[], "Attenuation dB"=[], "StepType"=enum."NewConnection"}, {"RF In/Out"=enum."Rx - RF Out", "TR Module 0-7"=62, "Polarization"=enum."Vertical", "PhaseShift deg"=[0.0, 5.625, 11.25, 16.875, 22.5, 28.125], "Attenuation dB"=[0.0, 0.5, 1.0, 1.5, 2.0, 2.5], "StepType"=enum."SweepTest"}, {"RF In/Out"=enum."Rx - RF Out", "TR Module 0-7"=63, "Polarization"=enum."Vertical", "PhaseShift deg"=[], "Attenuation dB"=[], "StepType"=enum."NewConnection"}, {"RF In/Out"=enum."Rx - RF Out", "TR Module 0-7"=63, "Polarization"=enum."Vertical", "PhaseShift deg"=[0.0, 5.625, 11.25, 16.875, 22.5, 28.125], "Attenuation dB"=[0.0, 0.5, 1.0, 1.5, 2.0, 2.5], "StepType"=enum."SweepTest"}, {"RF In/Out"=enum."Tx - RF In", "TR Module 0-7"=0, "Polarization"=enum."Vertical", "PhaseShift deg"=[], "Attenuation dB"=[], "StepType"=enum."Finish"}]
  in  "Phase three":T7={"StepType"=enum."Finish", "RF In/Out"=enum."Tx - RF In", "Module/Raster"=0, "Polarization"=enum."Vertical", "PhaseShift deg"=[], "Attenuation dB"=[], "Position"={"X mm"=0.0, "Y mm"=0.0, "Z mm"=0.0, "T deg"=0.0}, "Patch RF In/Out"=FALSE}
  in  "Phase two":T8
  # "IF Park & Measure\nTHEN\n   convert Phase2 sequence to phase 3\n   sequence as shown in this VI"
  # "#TBD save new typedefs"
  # "proposed:"
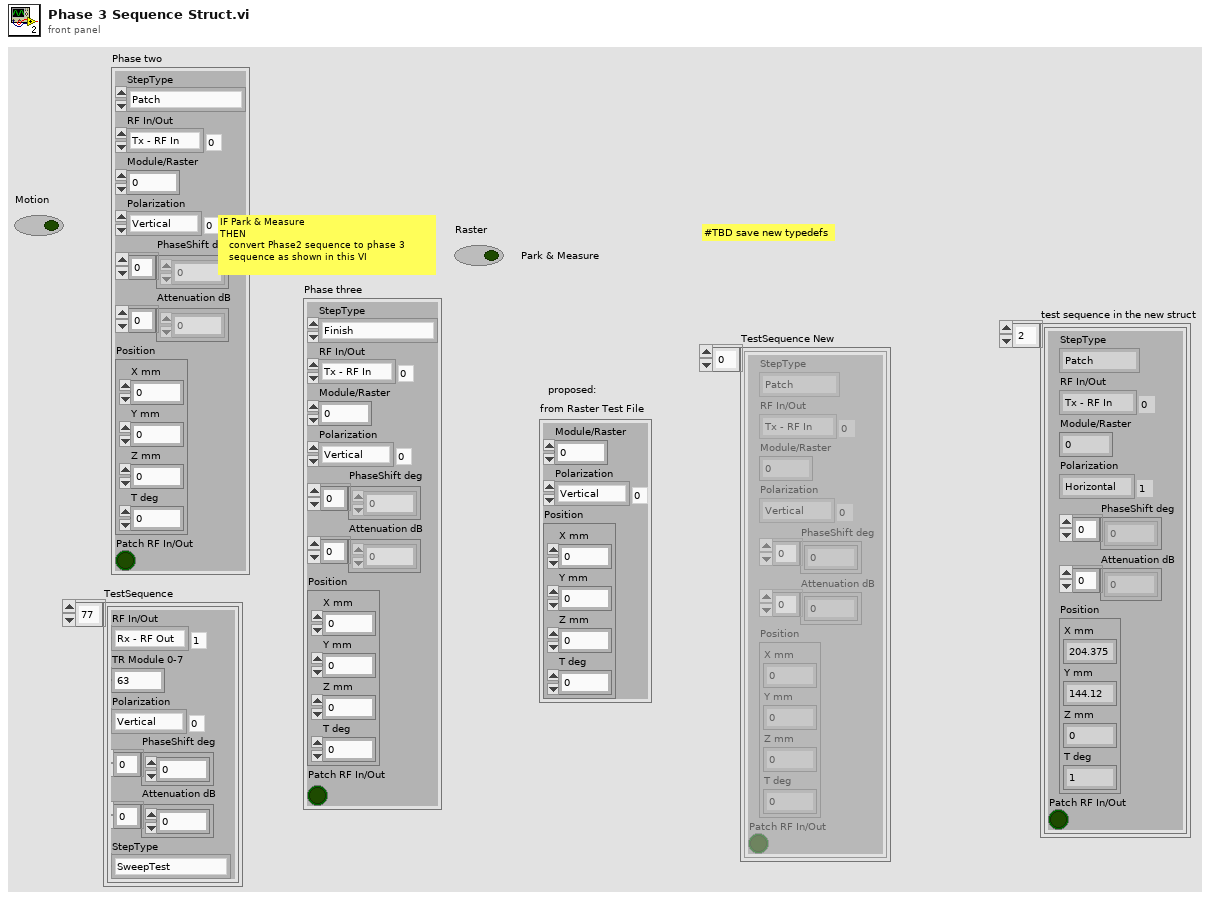
[diagram p1: front panel]
types:
  T1 = typedef "RF Direction.ctl" = enum16{"Tx - RF In", "Rx - RF Out"}
  T2 = typedef "PolarizationSelect.ctl" = enum16{"Vertical", "Horizontal"}
  T3 = cluster{"StepType":enum16{"Patch", "Motion", "SweepTest", "RasterTest", "Finish"}, "RF In/Out":T1, "Module/Raster":i32, "Polarization":T2, "PhaseShift deg":dbl[], "Attenuation dB":dbl[], "Position":cluster{"X mm":dbl, "Y mm":dbl, "Z mm":dbl, "T deg":dbl}, "Patch RF In/Out":bool}[]
  T4 = cluster{"Module/Raster":i32, "Polarization":T2, "Position":cluster{"X mm":dbl, "Y mm":dbl, "Z mm":dbl, "T deg":dbl}}
  T5 = typedef "TestStep-StepType.ctl" = cluster{"RF In/Out":T1, "TR Module 0-7":i32, "Polarization":T2, "PhaseShift deg":dbl[], "Attenuation dB":dbl[], "StepType":T6}
  T6 = typedef "TestStepTypes.ctl" = enum16{"NewConnection", "SweepTest", "Motion", "Finish"}
  T7 = cluster{"StepType":enum16{"Patch", "Motion", "SweepTest", "RasterTest", "Finish"}, "RF In/Out":T1, "Module/Raster":i32, "Polarization":T2, "PhaseShift deg":dbl[], "Attenuation dB":dbl[], "Position":cluster{"X mm":dbl, "Y mm":dbl, "Z mm":dbl, "T deg":dbl}, "Patch RF In/Out":bool}
  T8 = typedef "TestStep-StepType.ctl" = cluster{"StepType":T9, "RF In/Out":T1, "Module/Raster":i32, "Polarization":T2, "PhaseShift deg":dbl[], "Attenuation dB":dbl[], "Position":cluster{"X mm":dbl, "Y mm":dbl, "Z mm":dbl, "T deg":dbl}, "Patch RF In/Out":bool}
  T9 = typedef "TestStepTypes.ctl" = enum16{"Patch", "Motion", "SweepTest", "RasterTest", "Finish"}
  T10 = cluster{"X mm":dbl, "Y mm":dbl, "Z mm":dbl, "T deg":dbl}[]
  T11 = enum16{"Patch", "Motion", "SweepTest", "RasterTest", "Finish"}
  T12 = cluster{"X mm":dbl, "Y mm":dbl, "Z mm":dbl, "T deg":dbl}
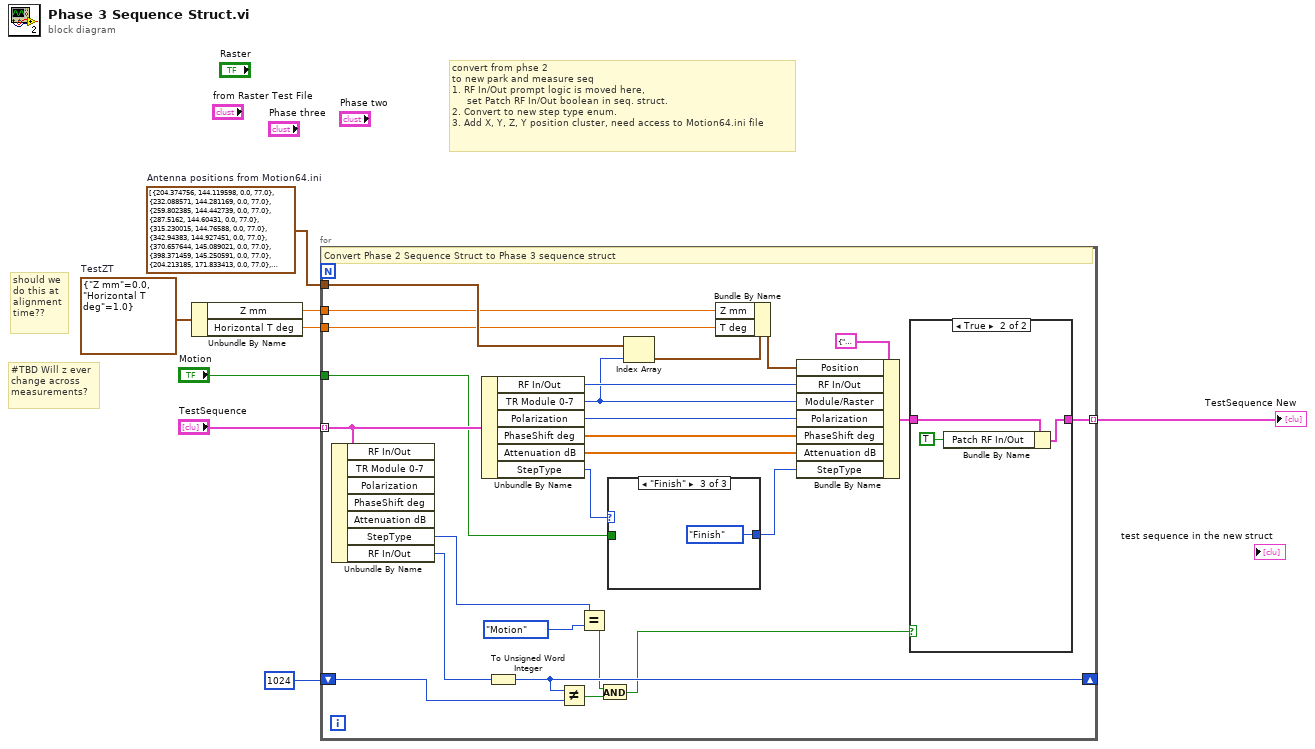
[diagram p0: block diagram]
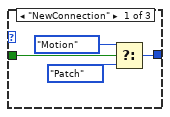
[diagram p3: hidden frame]
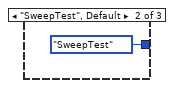
[diagram p4: hidden frame]
diagram:
  w3 = cluster{"Z mm":dbl, "Horizontal T deg":dbl} {"Z mm"=0.0, "Horizontal T deg"=1.0}  # TestZT
  w4 = T10 [{"X mm"=204.374756, "Y mm"=144.119598, "Z mm"=0.0, "T deg"=77.0}, {"X mm"=232.088571, "Y mm"=144.281169, "Z mm"=0.0, "T deg"=77.0}, {"X mm"=259.802385, "Y mm"=144.442739, "Z mm"=0.0, "T deg"=77.0}, {"X mm"=287.5162, "Y mm"=144.60431, "Z mm"=0.0, "T deg"=77.0}, {"X mm"=315.230015, "Y mm"=144.76588, "Z mm"=0.0, "T deg"=77.0}, {"X mm"=342.94383, "Y mm"=144.927451, "Z mm"=0.0, "T deg"=77.0}, {"X mm"=370.657644, "Y mm"=145.089021, "Z mm"=0.0, "T deg"=77.0}, {"X mm"=398.371459, "Y mm"=145.250591, "Z mm"=0.0, "T deg"=77.0}, {"X mm"=204.213185, "Y mm"=171.833413, "Z mm"=0.0, "T deg"=77.0}, {"X mm"=231.927, "Y mm"=171.994984, "Z mm"=0.0, "T deg"=77.0}, {"X mm"=259.640815, "Y mm"=172.156554, "Z mm"=0.0, "T deg"=77.0}, {"X mm"=287.35463, "Y mm"=172.318124, "Z mm"=0.0, "T deg"=77.0}, {"X mm"=315.068444, "Y mm"=172.479695, "Z mm"=0.0, "T deg"=77.0}, {"X mm"=342.782259, "Y mm"=172.641265, "Z mm"=0.0, "T deg"=77.0}, {"X mm"=370.496074, "Y mm"=172.802836, "Z mm"=0.0, "T deg"=77.0}, {"X mm"=398.209889, "Y mm"=172.964406, "Z mm"=0.0, "T deg"=77.0}, {"X mm"=204.051615, "Y mm"=199.547228, "Z mm"=0.0, "T deg"=77.0}, {"X mm"=231.76543, "Y mm"=199.708798, "Z mm"=0.0, "T deg"=77.0}, {"X mm"=259.479244, "Y mm"=199.870369, "Z mm"=0.0, "T deg"=77.0}, {"X mm"=287.193059, "Y mm"=200.031939, "Z mm"=0.0, "T deg"=77.0}, {"X mm"=314.906874, "Y mm"=200.19351, "Z mm"=0.0, "T deg"=77.0}, {"X mm"=342.620689, "Y mm"=200.35508, "Z mm"=0.0, "T deg"=77.0}, {"X mm"=370.334503, "Y mm"=200.51665, "Z mm"=0.0, "T deg"=77.0}, {"X mm"=398.048318, "Y mm"=200.678221, "Z mm"=0.0, "T deg"=77.0}, {"X mm"=203.890045, "Y mm"=227.261043, "Z mm"=0.0, "T deg"=77.0}, {"X mm"=231.603859, "Y mm"=227.422613, "Z mm"=0.0, "T deg"=77.0}, {"X mm"=259.317674, "Y mm"=227.584183, "Z mm"=0.0, "T deg"=77.0}, {"X mm"=287.031489, "Y mm"=227.745754, "Z mm"=0.0, "T deg"=77.0}, {"X mm"=314.745304, "Y mm"=227.907324, "Z mm"=0.0, "T deg"=77.0}, {"X mm"=342.459118, "Y mm"=228.068895, "Z mm"=0.0, "T deg"=77.0}, {"X mm"=370.172933, "Y mm"=228.230465, "Z mm"=0.0, "T deg"=77.0}, {"X mm"=397.886748, "Y mm"=228.392036, "Z mm"=0.0, "T deg"=77.0}, {"X mm"=203.728474, "Y mm"=254.974857, "Z mm"=0.0, "T deg"=77.0}, {"X mm"=231.442289, "Y mm"=255.136428, "Z mm"=0.0, "T deg"=77.0}, {"X mm"=259.156104, "Y mm"=255.297998, "Z mm"=0.0, "T deg"=77.0}, {"X mm"=286.869918, "Y mm"=255.459569, "Z mm"=0.0, "T deg"=77.0}, {"X mm"=314.583733, "Y mm"=255.621139, "Z mm"=0.0, "T deg"=77.0}, {"X mm"=342.297548, "Y mm"=255.782709, "Z mm"=0.0, "T deg"=77.0}, {"X mm"=370.011363, "Y mm"=255.94428, "Z mm"=0.0, "T deg"=77.0}, {"X mm"=397.725177, "Y mm"=256.10585, "Z mm"=0.0, "T deg"=77.0}, {"X mm"=203.566904, "Y mm"=282.688672, "Z mm"=0.0, "T deg"=77.0}, {"X mm"=231.280718, "Y mm"=282.850243, "Z mm"=0.0, "T deg"=77.0}, {"X mm"=258.994533, "Y mm"=283.011813, "Z mm"=0.0, "T deg"=77.0}, {"X mm"=286.708348, "Y mm"=283.173383, "Z mm"=0.0, "T deg"=77.0}, {"X mm"=314.422163, "Y mm"=283.334954, "Z mm"=0.0, "T deg"=77.0}, {"X mm"=342.135977, "Y mm"=283.496524, "Z mm"=0.0, "T deg"=77.0}, {"X mm"=369.849792, "Y mm"=283.658095, "Z mm"=0.0, "T deg"=77.0}, {"X mm"=397.563607, "Y mm"=283.819665, "Z mm"=0.0, "T deg"=77.0}, {"X mm"=203.405333, "Y mm"=310.402487, "Z mm"=0.0, "T deg"=77.0}, {"X mm"=231.119148, "Y mm"=310.564057, "Z mm"=0.0, "T deg"=77.0}, {"X mm"=258.832963, "Y mm"=310.725628, "Z mm"=0.0, "T deg"=77.0}, {"X mm"=286.546778, "Y mm"=310.887198, "Z mm"=0.0, "T deg"=77.0}, {"X mm"=314.260592, "Y mm"=311.048769, "Z mm"=0.0, "T deg"=77.0}, {"X mm"=341.974407, "Y mm"=311.210339, "Z mm"=0.0, "T deg"=77.0}, {"X mm"=369.688222, "Y mm"=311.371909, "Z mm"=0.0, "T deg"=77.0}, {"X mm"=397.402037, "Y mm"=311.53348, "Z mm"=0.0, "T deg"=77.0}, {"X mm"=203.243763, "Y mm"=338.116302, "Z mm"=0.0, "T deg"=77.0}, {"X mm"=230.957578, "Y mm"=338.277872, "Z mm"=0.0, "T deg"=77.0}, {"X mm"=258.671392, "Y mm"=338.439442, "Z mm"=0.0, "T deg"=77.0}, {"X mm"=286.385207, "Y mm"=338.601013, "Z mm"=0.0, "T deg"=77.0}, {"X mm"=314.099022, "Y mm"=338.762583, "Z mm"=0.0, "T deg"=77.0}, {"X mm"=341.812837, "Y mm"=338.924154, "Z mm"=0.0, "T deg"=77.0}, {"X mm"=369.526651, "Y mm"=339.085724, "Z mm"=0.0, "T deg"=77.0}, {"X mm"=397.240466, "Y mm"=339.247295, "Z mm"=0.0, "T deg"=77.0}]  # Antenna positions from Motion64.ini
  # "#TBD Will z ever\nchange across \nmeasurements?"
  # "should we\ndo this at\nalignment\ntime??"
  # "convert from phse 2\nto new park and measure seq\n1. RF In/Out prompt logic is moved here, \n     set Patch RF In/Out boolean in seq. struct.\n2. Convert to new step type enum.\n3. Add X, Y, Z, Y position cluster, need access to Motion64.ini file"
  n1 = Unbundle By Name(w3) -> ("Z mm"=w2:dbl, "Horizontal T deg"=w1:dbl)
  n2 = for {
    tunnel: "TestSequence" -> [w26] mode=indexing
    shift-right: [w30] -> _
    shift-left: u16 1024 -> [w31]
    tunnel: "Motion" -> [w20]
    tunnel: [w15] -> w5 mode=indexing
    tunnel: w4 -> [w14]
    tunnel: w2 -> [w10]
    tunnel: w1 -> [w9]
    # "Convert Phase 2 Sequence Struct to Phase 3 sequence struct"
    n3 = Unbundle By Name(w26) -> ("StepType"=w27:T6, "RF In/Out"=w32:T1)  [unwired: 5 out]
    n4 = Unbundle By Name(w26) -> ("RF In/Out"=w25:T1, "TR Module 0-7"=w13:i32, "Polarization"=w24:T2, "PhaseShift deg"=w23:dbl[], "Attenuation dB"=w22:dbl[], "StepType"=w21:T6)
    n5 = To Unsigned Word Integer(number=w32) -> (unsigned 16bit integer=w30:u16)
    n6 = Not Equal?(x=w30, y=w31) -> (x != y?=w29:bool)
    n7 = Equal?(x=w27, y=TestStepTypes."Motion" ("StepType")) -> (x = y?=w28:bool)
    n8 = And(x=w28, y=w29) -> (x .and. y?=w18:bool)
    n9 = case shown="\"Finish\"" w21 {
      tunnel: w20 -> [w39 _ _]
      tunnel: [w38 T11."SweepTest" ("StepType") T11."Finish" ("StepType")] -> w19
      frame "NewConnection" {
        n10 = Select(t=T11."Motion" ("StepType"), s=w39, f=T11."Patch" ("StepType")) -> (s? t:f=w38:T11)
      }
      frame "SweepTest", Default {
      }
      frame "Finish" {
      }
    }
    n11 = Index Array(array=w14, index=w13) -> (element=w12:T12)
    n12 = Bundle By Name(cluster=w12, "Z mm"=w10, "T deg"=w9) -> (w11:T12)
    n13 = Bundle By Name(cluster=T7 {"StepType"=enum."RasterTest", "RF In/Out"=enum."Tx - RF In", "Module/Raster"=0, "Polarization"=enum."Vertical", "PhaseShift deg"=[], "Attenuation dB"=[], "Position"={"X mm"=0.0, "Y mm"=0.0, "Z mm"=0.0, "T deg"=0.0}, "Patch RF In/Out"=FALSE} ("Phase three"), "Position"=w11, "RF In/Out"=w25, "Module/Raster"=w13, "Polarization"=w24, "PhaseShift deg"=w23, "Attenuation dB"=w22, "StepType"=w19) -> (w17:T7)
    n14 = case shown="True" w18 {
      tunnel: w17 -> [w34 w37]
      tunnel: [w34 w35] -> w15
      frame False {
      }
      frame True {
        n15 = Bundle By Name(cluster=w37, "Patch RF In/Out"=TRUE) -> (w35:T7)
      }
    }
  }
  "TestSequence New" <- w5
